vi "Raman.vi"() -> ()   [LabVIEW 2009]
uses:
  <instrlib>/Agilent ESG Series/Agilent ESG Series.lvlib
panel:
  in  "Amplitude (-135.00)":dbl=-135.0 format="%.2f"
  in  "Frequency (1000.0)":dbl=1000.0 format="%#.3g"
  in  "Stop Frequency":dbl[unit]=100000000.0
  out "error out":errorcluster {"code" format="%.0x"}
  in  "error in (no error)":errorcluster {"code" format="%.0x"}
  in  "VISA session":refnum<visa-resource-name>
  in  "Numeric":dbl
  in  "Number of Points":dbl=200.0
  in  "Increment":dbl[unit]
  in  "Start Frequency":dbl[unit]=100000000.0
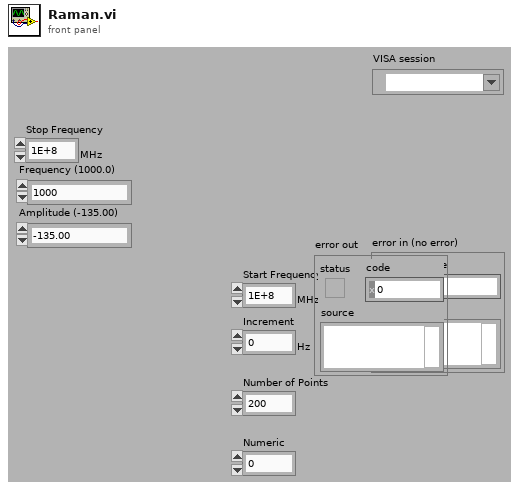
[diagram p1: front panel]
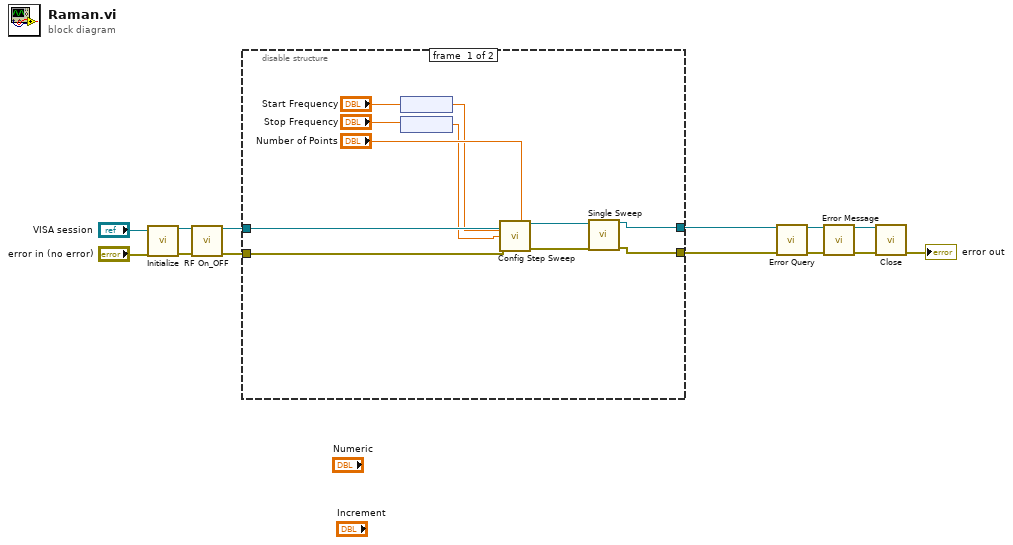
[diagram p0: block diagram]
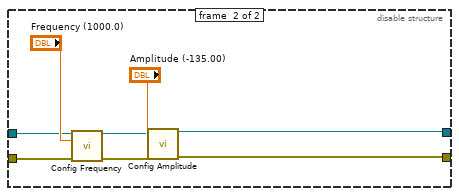
[diagram p2: hidden frame]
diagram:
  n1 = call <instrlib>:"Initialize.vi"("VISA Resource Name"="VISA session", "error in (no error)"="error in (no error)") -> ("VISA Resource Name Out"=w11:refnum<visa-resource-name>, "error out"=w10:errorcluster)  [unwired: 12 in]
  n2 = call <instrlib>:"RF On_OFF.vi"("VISA Resource Name"=w11, "error in (no error)"=w10) -> ("VISA Resource Name Out"=w4:refnum<visa-resource-name>, "error out"=w3:errorcluster)  [unwired: 12 in]
  n3 = disable-structure shown="Enabled" {
    disable-tunnel: w4 -> [w24 w30]
    disable-tunnel: w3 -> [w23 w29]
    disable-tunnel: [w15 w26] -> w2
    disable-tunnel: [w14 w25] -> w1
    frame #0 {
      n4 = node("Start Frequency") -> (w18:dbl)
      n5 = node("Stop Frequency") -> (w19:dbl)
      n6 = call <instrlib>:"Config Step Sweep.vi"("VISA Resource Name"=w24, "# Points (2)"="Number of Points", "Frequency Start (1000.00)"=w18, "Frequency Stop (1000.00)"=w19, "error in (no error)"=w23) -> ("VISA Resource Name Out"=w17:refnum<visa-resource-name>, "error out"=w16:errorcluster)  [unwired: 9 in]
      n7 = call <instrlib>:"Single Sweep.vi"("VISA Resource Name"=w17, "error in (no error)"=w16) -> ("VISA Resource Name Out"=w15:refnum<visa-resource-name>, "error out"=w14:errorcluster)  [unwired: 12 in]
    }
    frame #1 {
      n8 = call <instrlib>:"Config Frequency.vi"("VISA Resource Name"=w30, "Frequency (1000.0)"="Frequency (1000.0)", "error in (no error)"=w29) -> ("VISA Resource Name Out"=w28:refnum<visa-resource-name>, "error out"=w27:errorcluster)  [unwired: 11 in]
      n9 = call <instrlib>:"Config Amplitude.vi"("VISA Resource Name"=w28, "Amplitude (-135.00)"="Amplitude (-135.00)", "error in (no error)"=w27) -> ("VISA Resource Name Out"=w26:refnum<visa-resource-name>, "error out"=w25:errorcluster)  [unwired: 11 in]
    }
  }
  n10 = call <instrlib>:"Error Query.vi"("VISA Resource Name"=w2, "error in (no error)"=w1) -> ("VISA Resource Name Out"=w6:refnum<visa-resource-name>, "error out"=w9:errorcluster)  [unwired: 10 in, 2 out]
  n11 = call <instrlib>:"Error Message.vi"("VISA Resource Name"=w6, "error in (no error)"=w9) -> ("VISA Resource Name Out"=w7:refnum<visa-resource-name>, "error out"=w8:errorcluster)  [unwired: 9 in, 3 out]
  n12 = call <instrlib>:"Close.vi"("VISA Resource Name"=w7, "error in (no error)"=w8) -> ("error out"=→"error out":errorcluster)  [unwired: 13 in]
